vi "Log Value to File.vi"(8 "error in (no error)":errorcluster, 10 "Data Record":T1, 11 "Datalogger Actor in":refnum<class "Datalogger Actor.lvclass">) -> (0 "error out":errorcluster, 3 "Datalogger Actor out":refnum<class "Datalogger Actor.lvclass">)   [LabVIEW 2018, in "Datalogger Actor.lvlib" / "Datalogger Actor.lvclass"]
uses:
  Datalogger Actor.lvclass
  Data Record Control.ctl
  Datalogger Actor.lvclass/Datalogger Actor.ctl
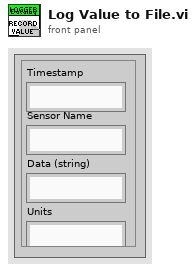
[diagram p1: front panel]
types:
  T1 = typedef "Datalogger Actor.lvlib/Datalogger Actor.lvclass/Data Record Control.ctl" = cluster{"Timestamp":string, "Sensor Name":string, "Data (string)":string, "Units":string}
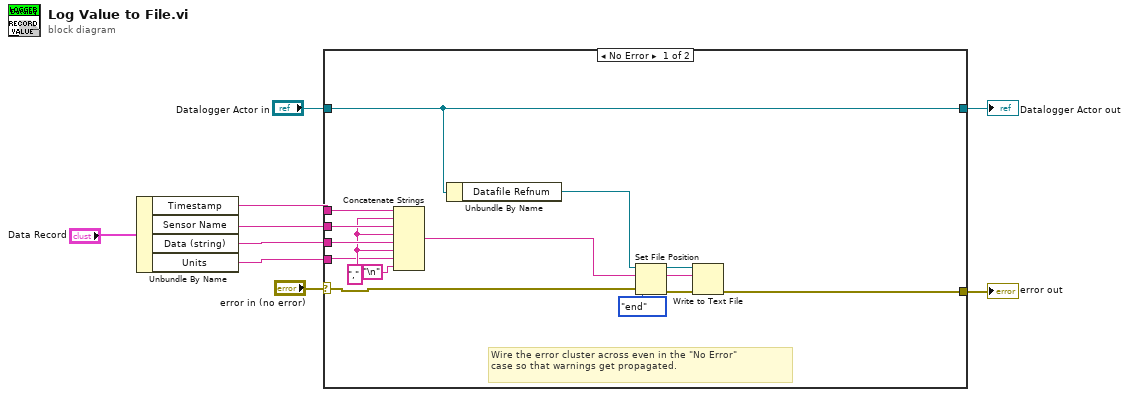
[diagram p0: block diagram]
diagram:
  n1 = Unbundle By Name("Data Record") -> ("Timestamp"=w3:string, "Sensor Name"=w2:string, "Data (string)"=w5:string, "Units"=w4:string)
  n2 = case shown="No Error" "error in (no error)" {
    selector: "error in (no error)" -> [w14 w25]
    tunnel: [w23 w25] -> w8
    tunnel: [w21 w24] -> w6
    tunnel: "Datalogger Actor in" -> [w21 w24]
    tunnel: w5 -> [w19 _]
    tunnel: w4 -> [w16 _]
    tunnel: w3 -> [w22 _]
    tunnel: w2 -> [w20 _]
    frame No Error {
      w18 = "," ("string")
      # "Wire the error cluster across even in the \"No Error\"\ncase so that warnings get propagated."
      n3 = Concatenate Strings(w22, w18, w20, w18, w19, w18, w16, "\n") -> (w11:string)
      n4 = Unbundle By Name(w21) -> ("Datafile Refnum"=w15:refnum<file>)
      n5 = Set File Position(refnum=w15, from (0:start)=enum16{"start", "end", "current"}."end", error in=w14) -> (refnum out=w13:refnum<file>, error out=w12:errorcluster)  [unwired: 1 in]
      n6 = Write to Text File(file (use dialog)=w13, text=w11, error in=w12) -> (error out=w23:errorcluster)  [unwired: 1 in, 2 out]
    }
    frame Error {
    }
  }
  "error out" <- w8
  "Datalogger Actor out" <- w6
